vi "Pockels Cal-Parse cal table strings.vi"(9 "Processing Type (Interpolate)":T1, 11 "SINGLE CAL SET (inc. headers & info)":string[][](array[string])=[["Cal Wavelength", ""], ["820", ""], ["Prism 1:", "2039"], ["Prism 2:", "1953"], ["Pockels offset:", "199"], ["Zoom:", "12"], ["Dwell time:", "0.4"], ["Cal subset indexes", ""], ["0", "14"], ["Cal data", ""], ["Pockels V", "No objective"], ["0", "0"], ["0.1", "2.8"], ["0.2", "9.8"], ["0.3", "21.4"], ["0.4", "37.1"], ["0.5", "56.1"], ["0.6", "77.7"], ["0.7", "101"], ["0.8", "125"], ["0.9", "148"], ["1", "169"], ["1.1", "188"], ["1.2", "204"], ["1.3", "215"], ["1.4", "222"], ["1.5", "225"], ["1.6", "222"], ["1.7", "214"], ["1.8", "202"], ["1.9", "187"], ["2", "152"]]) -> (0 "error out":errorcluster, 1 "Pockels Cal data":dbl[][](array[numeric]), 2 "Cal subset indexes":T3={"Start point index"=0, "End point index"=11}, 3 "SINGLE CAL SET / Pockels Cal table (inc. headers & info)":string[][](array[string]), 4 "Cal data header":string[](array[string]), 5 "Cal conditions":T2)   [LabVIEW 2020]
uses:
  Typedefs/Pockels cal conditions cluster.ctl
  Typedefs/Pockels cal processing type.ctl
panel:
  out "Pockels Cal data only (strings)":string[][](array[string])
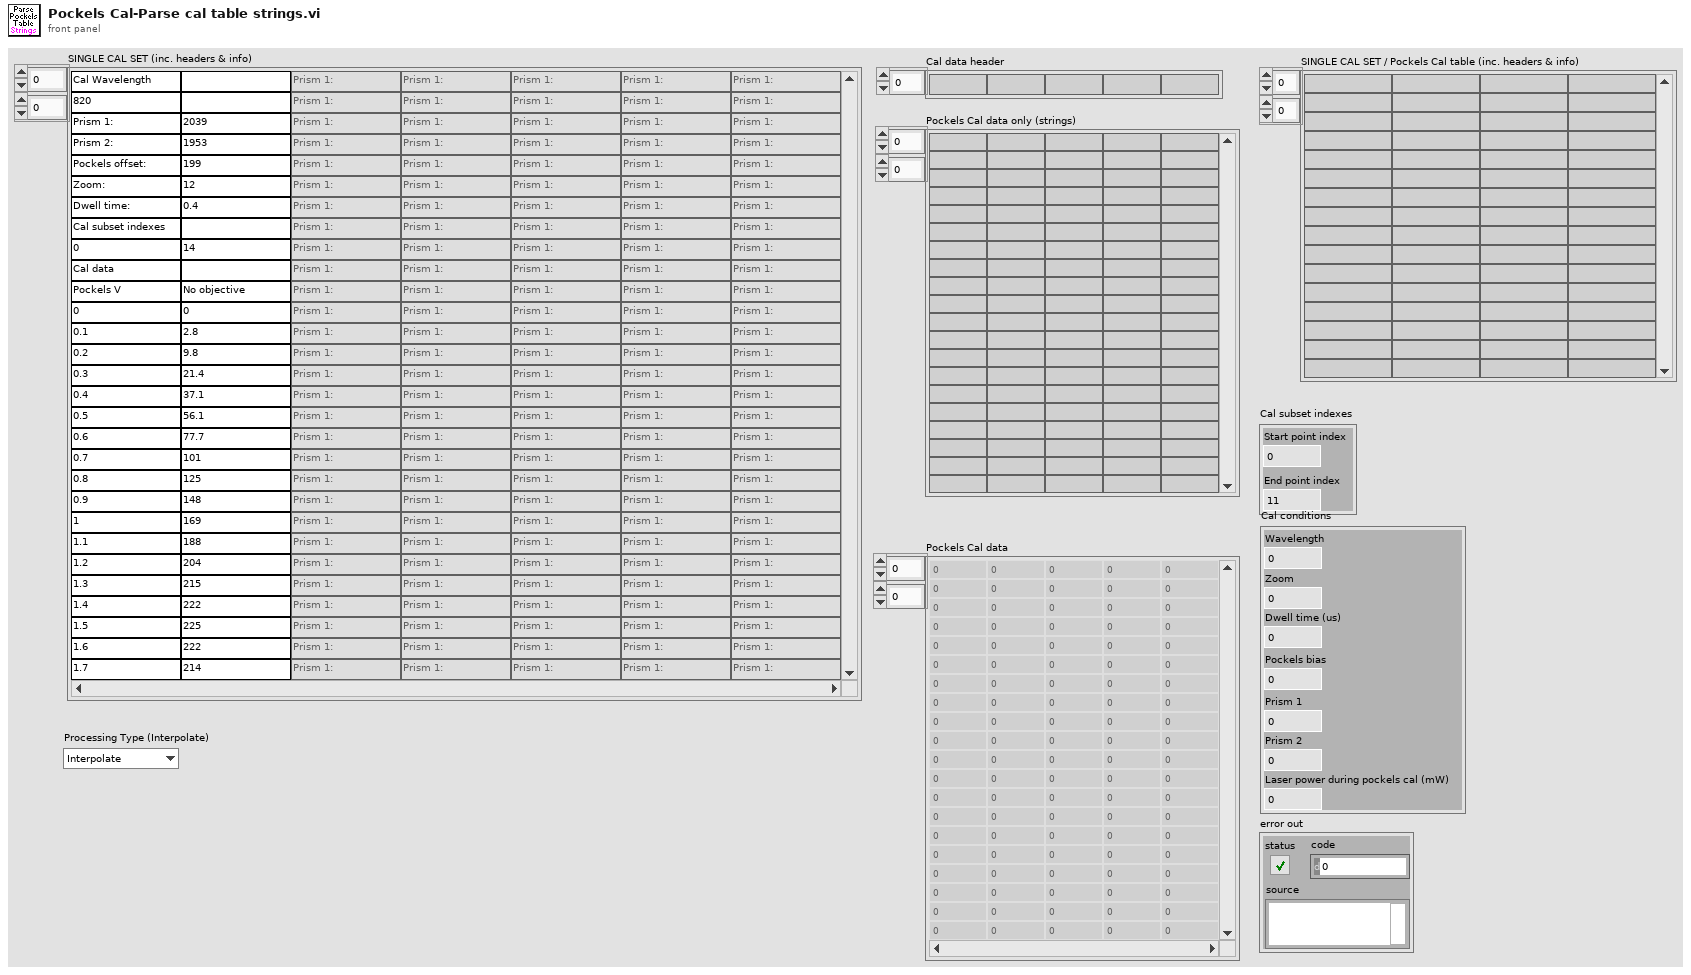
[diagram p1: front panel]
types:
  T1 = typedef "Pockels cal processing type.ctl" = enum16{"Interpolate", "Condense"}
  T2 = typedef "Pockels cal conditions cluster.ctl" = cluster{"Wavelength":u16, "Zoom":u8, "Dwell time (us)":dbl, "Pockels bias":i16, "Prism 1":u16, "Prism 2":u16, "Laser power during pockels cal (mW)":u16}
  T3 = cluster{"Start point index":i32, "End point index":i32}
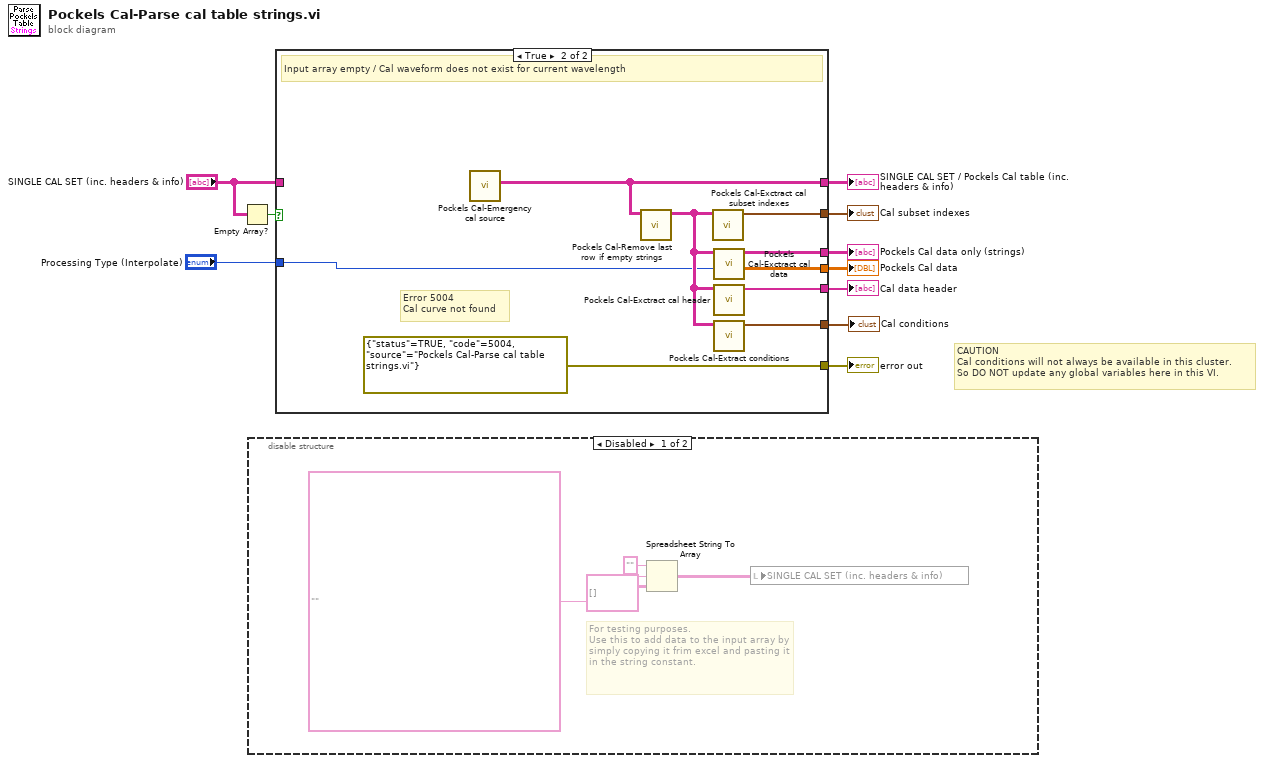
[diagram p0: block diagram]
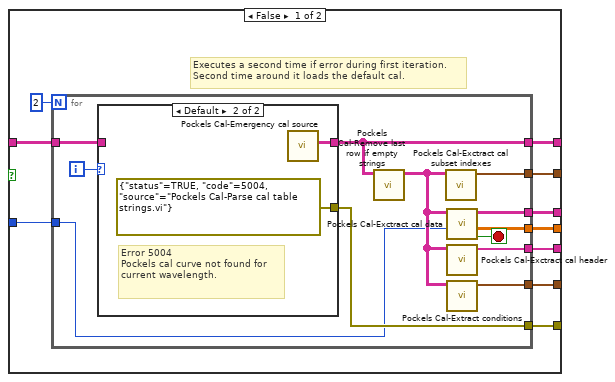
[diagram p2: hidden frame]
diagram:
  # "CAUTION\nCal conditions will not always be available in this cluster.\nSo DO NOT update any global variables here in this VI."
  n1 = Empty Array?(array="SINGLE CAL SET (inc. headers & info)") -> (empty?=w5:bool)
  n2 = disable-structure shown="Disabled" {
    frame Disabled {
      # "For testing purposes.\nUse this to add data to the input array by simply copying it frim excel and pasting it in the string constant."
      n3 = Spreadsheet String To Array(format string="", spreadsheet string="" ("format string"), array type (2D Dbl)=string[][] []) -> (array=w12:string[][])  [unwired: 1 in]
      n4 = local write "SINGLE CAL SET (inc. headers & info)"(w12) -> ()
    }
    frame Enabled {
    }
  }
  n5 = case shown="True" w5 {
    tunnel: [w24 w48] -> w10
    tunnel: "SINGLE CAL SET (inc. headers & info)" -> [w23 _]
    tunnel: [w22 w47] -> w9
    tunnel: [w21 w46] -> w8
    tunnel: [w20 w45] -> w7
    tunnel: [w18 w44] -> w6
    tunnel: [w17 errorcluster {"status"=TRUE, "code"=5004, "source"="Pockels Cal-Parse cal table strings.vi"} ("error out")] -> w3
    tunnel: [w16 w42] -> w2
    tunnel: "Processing Type (Interpolate)" -> [w15 w40]
    frame False {
      # "Executes a second time if error during first iteration.\nSecond time around it loads the default cal."
      n6 = for {
        N: 2 -> [_]
        tunnel: [w36] -> w24
        tunnel: w23 -> [w30]
        tunnel: [w35] -> w22
        tunnel: [w34] -> w21
        tunnel: [w33] -> w20
        tunnel: [w29] -> w18
        tunnel: [w28] -> w17
        tunnel: [w26] -> w16
        tunnel: w15 -> [w25]
        i -> [w31]
        stop <- w32 stop-if-true
        n7 = case shown="Default" w31 {
          tunnel: w30 -> [w37 _]
          tunnel: [w37 w39] -> w29
          tunnel: [_ errorcluster {"status"=TRUE, "code"=5004, "source"="Pockels Cal-Parse cal table strings.vi"} ("error out")] -> w28
          frame 0 {
          }
          frame Default {
            # "Error 5004\nPockels cal curve not found for current wavelength."
            n8 = call "Pockels Cal-Emergency cal source.vi"() -> ("SINGLE CAL SET (inc. headers & info)"=w39:string[][])  [unwired: 11 in]
          }
        }
        n9 = call "Pockels Cal-Remove last row if empty strings.vi"("Pockels Cal table"=w29) -> ("Pockels Cal table (inc. header line)"=w27:string[][])  [unwired: 10 in]
        n10 = call "Pockels Cal-Exctract cal subset indexes.vi"("Pockels Cal table"=w27) -> ("Cal subset indexes"=w36:T3)  [unwired: 10 in]
        n11 = call "Pockels Cal-Exctract cal data.vi"("Processing Type (Interpolate)"=w25, "Pockels Cal table (full)"=w27) -> ("OK"=w32:bool, "Pockels Cal data (DBL)"=w34:dbl[][], "Pockels Cal data (strings)"=w35:string[][])  [unwired: 6 in, 1 out]
        n12 = call "Pockels Cal-Exctract cal header.vi"("Pockels Cal table (full)"=w27) -> ("Cal data header"=w33:string[])  [unwired: 10 in]
        n13 = call "Pockels Cal-Extract conditions.vi"("Pockels Cal table (full)"=w27) -> ("Pockels cal conditions"=w26:T2)  [unwired: 8 in, 2 out]
      }
    }
    frame True {
      # "Error 5004\nCal curve not found"
      # "Input array empty / Cal waveform does not exist for current wavelength"
      n14 = call "Pockels Cal-Emergency cal source.vi"() -> ("SINGLE CAL SET (inc. headers & info)"=w44:string[][])  [unwired: 11 in]
      n15 = call "Pockels Cal-Remove last row if empty strings.vi"("Pockels Cal table"=w44) -> ("Pockels Cal table (inc. header line)"=w43:string[][])  [unwired: 10 in]
      n16 = call "Pockels Cal-Exctract cal subset indexes.vi"("Pockels Cal table"=w43) -> ("Cal subset indexes"=w48:T3)  [unwired: 10 in]
      n17 = call "Pockels Cal-Exctract cal data.vi"("Processing Type (Interpolate)"=w40, "Pockels Cal table (full)"=w43) -> ("Pockels Cal data (DBL)"=w46:dbl[][], "Pockels Cal data (strings)"=w47:string[][])  [unwired: 6 in, 2 out]
      n18 = call "Pockels Cal-Exctract cal header.vi"("Pockels Cal table (full)"=w43) -> ("Cal data header"=w45:string[])  [unwired: 10 in]
      n19 = call "Pockels Cal-Extract conditions.vi"("Pockels Cal table (full)"=w43) -> ("Pockels cal conditions"=w42:T2)  [unwired: 8 in, 2 out]
    }
  }
  "Pockels Cal data only (strings)" <- w9
  "Pockels Cal data" <- w8
  "Cal subset indexes" <- w10
  "Cal data header" <- w7
  "SINGLE CAL SET / Pockels Cal table (inc. headers & info)" <- w6
  "error out" <- w3
  "Cal conditions" <- w2
